vi "Read from Hardware.vi"(8 "error in":errorcluster, 10 "values in":dbl[](array[numeric]), 11 "logging execution unit in":refnum<class "Logging Execution Unit.lvclass">) -> (0 "error out":errorcluster, 2 "values out":dbl[](array[numeric]), 3 "logging execution unit out":refnum<class "Logging Execution Unit.lvclass">)   [LabVIEW 2020, in "Ballard MIL-STD-1553 Engine.lvlib" / "Implementation.lvlib" / "Logging Execution Unit.lvclass"]
uses:
  Logging Execution Unit.lvclass
  C:/Users/nitest/Desktop/Git 2020/niveristand-ballard-milStd1553-custom-device/Source/Custom Device Support/Engine/Implementation/Execution Unit/Execution Unit.lvclass
  Execution Unit/Execution Unit.lvclass/Execution Unit.ctl
  Logging Execution Unit.lvclass/Logging Execution Unit.ctl
  Custom Device/Write Error to System Log.vi/ca55ed61-c1f5-4d13-8aef-490b87d2cf89.vi
  <vilib>/NI VeriStand/Custom Device Tools/Custom Device Utility Library/NI VeriStand - Print Debug Line.vi
  <instrlib>/BTICardLib/BTICardLV.lvlib
  Execution Unit/Execution Unit.lvclass
  Logging/Word Logging/Word Logging.lvlib
  Custom Device/Custom Device.lvlib
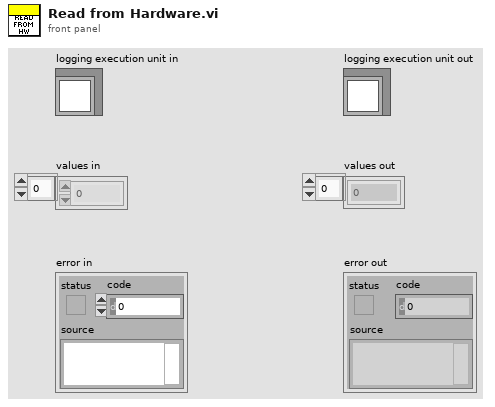
[diagram p1: front panel]
types:
  T1 = typedef "Ballard MIL-STD-1553 Engine.lvlib/Custom Device.lvlib/Hardware Handles.ctl" = cluster{"core handle":u64, "core reader handle":u64, "channel handles":u64[]}
  T2 = typedef "BTICardLV.lvlib/1553 Record.ctl" = cluster{"type":u16, "count":u16, "timestamp":u32, "activity":u16, "error":u16, "cwd1":u16, "cwd2":u16, "swd1":u16, "swd2":u16, "datacount":u16, "data":u16[], "timestamph":u32, "resptime1":u16, "resptime2":u16}
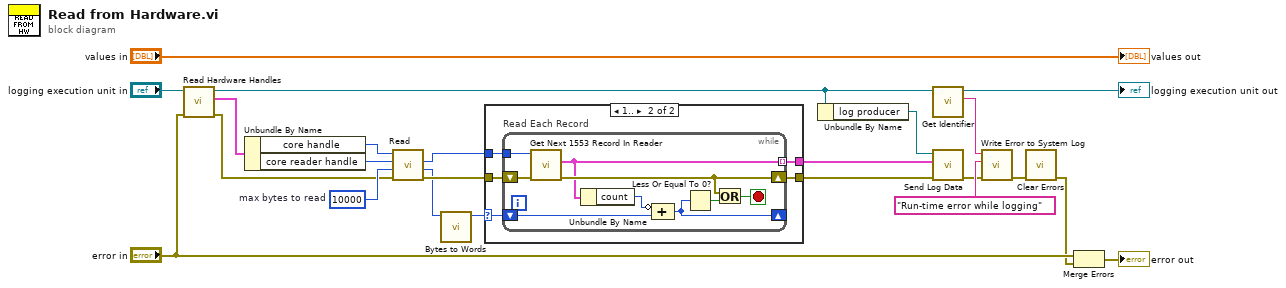
[diagram p0: block diagram]
diagram:
  w23 = 10000  # max bytes to read
  n1 = call "Read Hardware Handles.vi"("error in"="error in", "Execution Unit in"="logging execution unit in") -> ("error out"=w22:errorcluster, "hardware handles"=w21:T1, "Execution Unit out"=w7:refnum<class "Logging Execution Unit.lvclass">)  [unwired: 7 in]
  n2 = Unbundle By Name(w21) -> ("core handle"=w18:u64, "core reader handle"=w17:u64)
  n3 = call <instrlib>:"Read.vi"("error in (no error)"=w22, "max bytes to read"=w23, "core reader handle in"=w17, "core handle in"=w18) -> ("error out"=w20:errorcluster, "bytes read"=w15:i32, "core reader handle out"=w19:u64)  [unwired: 4 in, 1 out]
  n4 = call "Bytes to Words.vi"("bytes"=w15) -> ("U16 words"=w16:u16)  [unwired: 10 in]
  n5 = case shown="1.." w16 {
    selector: w16 -> [_ w25]
    tunnel: w20 -> [w24 w29]
    tunnel: [w24 w28] -> w10
    tunnel: w19 -> [_ w27]
    tunnel: [_ w26] -> w13
    frame Default {
    }
    frame 1.. {
      n6 = while "Read Each Record" {
        tunnel: w27 -> [w38]
        tunnel: [w35] -> w26 mode=indexing
        shift-right: [w36] -> w28
        shift-left: w29 -> [w37]
        shift-right: [w33] -> _
        shift-left: w25 -> [w34]
        stop <- w31 stop-if-true
        n7 = call <instrlib>:"Get Next 1553 Record In Reader.vi"("error in (no error)"=w37, "core reader handle in"=w38) -> ("error out"=w36:errorcluster, "record out"=w35:T2)  [unwired: 7 in, 1 out]
        n8 = Unbundle By Name(w35) -> ("count"=w30:u16)
        n9 = Compound Arithmetic op=ADD(invert w30, w34) -> (w33:u16)
        n10 = Less Or Equal To 0?(x=w33) -> (x <= 0?=w32:bool)
        n11 = Or(x=w36, y=w32) -> (x .or. y?=w31:bool)
      }
    }
  }
  n12 = Unbundle By Name(w7) -> ("log producer"=w12:refnum<class "Log Producer.lvclass">)
  n13 = call-dynamic "Get Identifier.vi"("Execution Unit Implementation in"=w7) -> ("Identifier"=w4:string, "Execution Unit Implementation out"=→"logging execution unit out":refnum<class "Logging Execution Unit.lvclass">)  [unwired: 8 in, 1 out]
  n14 = call "Send Log Data.vi"("error in"=w10, "Data"=w13, "Producer in"=w12) -> ("error out"=w5:errorcluster)  [unwired: 7 in, 1 out]
  n15 = call "Write Error to System Log.vi"("error in"=w5, "message"="Run-time error while logging", "identifier"=w4) -> ("error out"=w9:errorcluster)  [unwired: 8 in]
  n16 = call <vilib>:"Clear Errors.vi"("error in (no error)"=w9) -> ("error out"=w2:errorcluster)  [unwired: 5 in, 1 out]
  n17 = Merge Errors("error in", w2) -> (→"error out":errorcluster)
  "values out" <- "values in"
